vi "PH_SHS_Analysis_Statistician.PC Clear Data.vi"(0 "i ref in":refnum<vi>, 5 "error IO":errorcluster) -> (14 "i ref out":refnum<vi>, 19 "error out":errorcluster)   [LabVIEW 2014, in "PH_SHS_Analysis_Statistician.lvlib"]
uses:
  PH_SHS_Analysis_Statistician.lvlib
  PH_SHS_Analysis/PH_SHS_Analysis.Zernike Dataset.ctl
  PH_StatusHandler/PH_StatusHandler.Status.ctl
  PH_SHS_Analysis/PH_SHS_Analysis.Zernike Coefficients.ctl
  PH_Common/PH_Common.lvlib
  PH_SHS_Analysis/PH_SHS_Analysis.lvlib
  PH_StatusHandler/PH_StatusHandler.lvlib
panel:
  in  "Empty Data":T1[](array[typedef]) {"State" items=["no info", "off/false/out", "on/true/in", "Failure", "Alarm", "Status 1", "Status 2", "Status 3"]; "Zernicke Coefficients"."2nd Spherical" scale=-2.0..2.0 scale format="%.2f"; "Zernicke Coefficients"."2nd Coma y" scale=-2.0..2.0 scale format="%.2f"; "Zernicke Coefficients"."2nd Coma x" scale=-2.0..2.0 scale format="%.2f"; "Zernicke Coefficients"."2nd Astig 45°" scale=-2.0..2.0 scale format="%.2f"; "Zernicke Coefficients"."2nd Astig 0°" scale=-2.0..2.0 scale format="%.2f"; "Zernicke Coefficients"."Trefoil 30°" scale=-2.0..2.0 scale format="%.2f"; "Zernicke Coefficients"."Trefoil 0°" scale=-2.0..2.0 scale format="%.2f"; "Zernicke Coefficients"."Spherical" scale=-2.0..2.0 scale format="%.2f"; "Zernicke Coefficients"."Coma y" scale=-2.0..2.0 scale format="%.2f"; "Zernicke Coefficients"."Coma x" scale=-2.0..2.0 scale format="%.2f"; "Zernicke Coefficients"."Astig 45°" scale=-2.0..2.0 scale format="%.2f"; "Zernicke Coefficients"."Astig 0°" scale=-2.0..2.0 scale format="%.2f"; "Zernicke Coefficients"."Defocus" scale=-2.0..2.0 scale format="%.2f"; "Zernicke Coefficients"."Tilt y" scale=-2.0..2.0 scale format="%.2f"; "Zernicke Coefficients"."Tilt x" scale=-2.0..2.0 scale format="%.2f"}
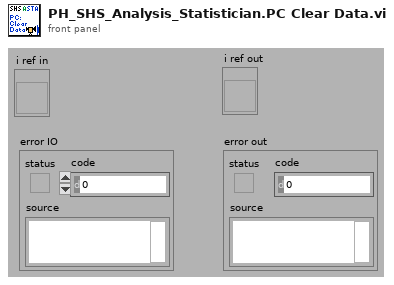
[diagram p1: front panel]
types:
  T1 = typedef "PH_SHS_Analysis.lvlib/PH_SHS_Analysis.Zernike Dataset.ctl" = cluster{"State":T2, "Time Stamp":timestamp, "PtV [lambda]":dbl, "Zernicke Coefficients":T3}
  T2 = typedef "PH_StatusHandler.lvlib/PH_StatusHandler.Status.ctl" = i16
  T3 = typedef "PH_SHS_Analysis.lvlib/PH_SHS_Analysis.Zernike Coefficients.ctl" = cluster{"Tilt x":dbl, "Tilt y":dbl, "Defocus":dbl, "Astig 0°":dbl, "Astig 45°":dbl, "Coma x":dbl, "Coma y":dbl, "Spherical":dbl, "Trefoil 0°":dbl, "Trefoil 30°":dbl, "2nd Astig 0°":dbl, "2nd Astig 45°":dbl, "2nd Coma x":dbl, "2nd Coma y":dbl, "2nd Spherical":dbl}
  T4 = typedef "PH_SHS_Analysis_Statistician.lvlib/PH_SHS_Analysis_Statistician.i attribute.ctl" = cluster{"GUI Refs ":cluster{"Status":refnum<vi>, "Result Graph":refnum<vi>, "Mean Data 1":refnum<vi>, "Std Dev Data 1":refnum<vi>, "Mean Data 2":refnum<vi>, "Std Dev Data 2":refnum<vi>, "Mean Data 3":refnum<vi>, "Std Dev Data 3":refnum<vi>, "Dummy Mean":refnum<vi>, "Dummy Std Dev":refnum<vi>, "Export Data":refnum<vi>, "Data 1":refnum<vi>, "Data 2":refnum<vi>, "Data 3":refnum<vi>, "Stat or Trend":refnum<vi>, "Delete":refnum<vi>, "Analyzer":refnum<vi>, "Current Zernike Coefficients":refnum<vi>, "PtV [Lambda]":refnum<vi>, "sample length":refnum<vi>}, "Analyzer":string, "Stat or Trend":bool, "Data 1":i16, "Data 2":i16, "Data 3":i16, "Data":T1[], "sample length":i32, "Datasets strored":i32, "Dataarray Size":i32}
  T5 = cluster{"Tilt x":dbl, "Tilt y":dbl, "Defocus":dbl, "Astig 0°":dbl, "Astig 45°":dbl, "Coma x":dbl, "Coma y":dbl, "Spherical":dbl, "Trefoil 0°":dbl, "Trefoil 30°":dbl, "2nd Astig 0°":dbl, "2nd Astig 45°":dbl, "2nd Coma x":dbl, "2nd Coma y":dbl, "2nd Spherical":dbl}
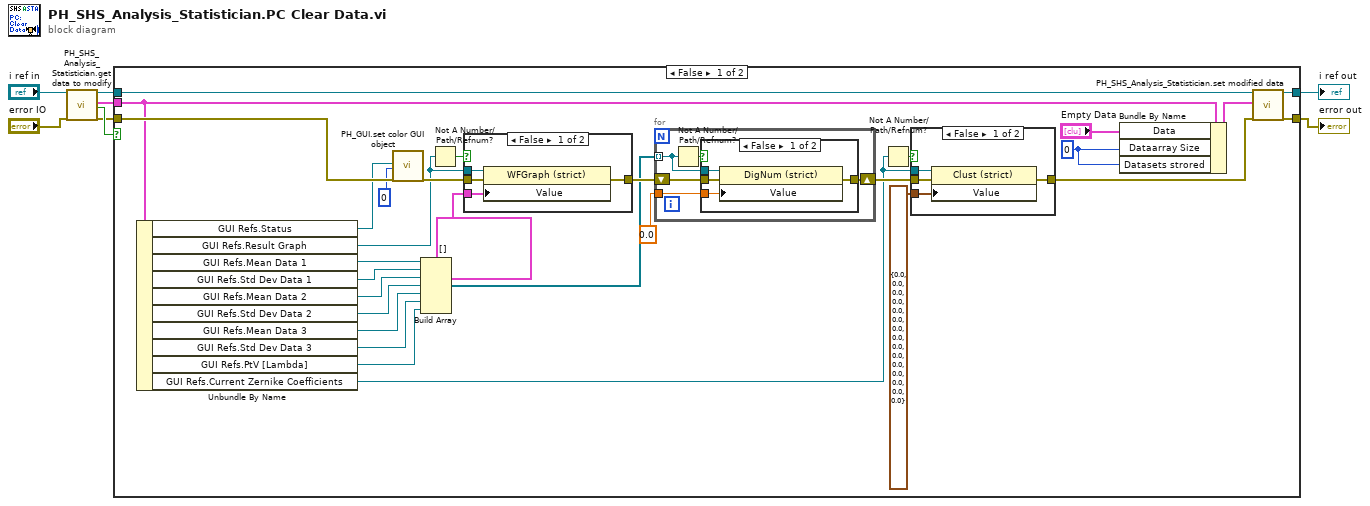
[diagram p0: block diagram]
diagram:
  n1 = call "PH_SHS_Analysis_Statistician.get data to modify.vi"("i ref in"="i ref in", "error in (no error)"="error IO") -> ("i ref out"=w5:refnum<vi>, "i attribute"=w8:T4, "timed out"=w7:bool, "error out"=w2:errorcluster)  [unwired: 14 in]
  n2 = case shown="False" w7 {
    tunnel: w2 -> [w37 w58]
    tunnel: [w36 w58] -> w3
    tunnel: w5 -> [w35 w59]
    tunnel: [w34 w59] -> w6
    tunnel: w8 -> [w31 _]
    frame False {
      w9 = 0 ("sample length")
      n3 = Unbundle By Name(w31) -> ("GUI Refs.Status"=w29:refnum<vi>, "GUI Refs.Result Graph"=w27:refnum<vi>, "GUI Refs.Mean Data 1"=w23:refnum<vi>, "GUI Refs.Std Dev Data 1"=w20:refnum<vi>, "GUI Refs.Mean Data 2"=w19:refnum<vi>, "GUI Refs.Std Dev Data 2"=w18:refnum<vi>, "GUI Refs.Mean Data 3"=w17:refnum<vi>, "GUI Refs.Std Dev Data 3"=w16:refnum<vi>, "GUI Refs.PtV [Lambda]"=w15:refnum<vi>, "GUI Refs.Current Zernike Coefficients"=w11:refnum<vi>)
      n4 = call "PH_GUI.set color GUI object.vi"("GUI object Ref"=w29, "State"=0, "error in (no error)"=w37) -> ("error out"=w30:errorcluster)  [unwired: 16 in]
      n5 = Build Array(w23, w20, w19, w18, w17, w16, w15) -> (w22:refnum<vi>[])
      n6 = Not A Number/Path/Refnum?(number/path/refnum=w27) -> (NaN/Path/Refnum?=w26:bool)
      n7 = case shown="False" w26 {
        tunnel: w30 -> [w56 w57]
        tunnel: [w55 w57] -> w24
        tunnel: w27 -> [w54 _]
        tunnel: cluster{dbl[], dbl[]}[] [] ("Value") -> [w53 _]
        frame False {
          n8 = property class="WFGraph (strict)"(reference=w54, error in=w56, "Value"=w53) -> (error out=w55:errorcluster)  [unwired: 1 out]
        }
        frame True {
        }
      }
      n9 = for {
        shift-right: [w45] -> w13
        shift-left: w24 -> [w46]
        tunnel: w22 -> [w44] mode=indexing
        tunnel: 0.0 ("Value") -> [w43]
        n10 = Not A Number/Path/Refnum?(number/path/refnum=w44) -> (NaN/Path/Refnum?=w47:bool)
        n11 = case shown="False" w47 {
          tunnel: w46 -> [w51 w52]
          tunnel: [w50 w52] -> w45
          tunnel: w44 -> [w49 _]
          tunnel: w43 -> [w48 _]
          frame False {
            n12 = property class="DigNum (strict)"(reference=w49, error in=w51, "Value"=w48) -> (error out=w50:errorcluster)  [unwired: 1 out]
          }
          frame True {
          }
        }
      }
      n13 = Not A Number/Path/Refnum?(number/path/refnum=w11) -> (NaN/Path/Refnum?=w14:bool)
      n14 = case shown="False" w14 {
        tunnel: w13 -> [w41 w42]
        tunnel: [w40 w42] -> w12
        tunnel: w11 -> [w39 _]
        tunnel: T5 {"Tilt x"=0.0, "Tilt y"=0.0, "Defocus"=0.0, "Astig 0°"=0.0, "Astig 45°"=0.0, "Coma x"=0.0, "Coma y"=0.0, "Spherical"=0.0, "Trefoil 0°"=0.0, "Trefoil 30°"=0.0, "2nd Astig 0°"=0.0, "2nd Astig 45°"=0.0, "2nd Coma x"=0.0, "2nd Coma y"=0.0, "2nd Spherical"=0.0} ("Value") -> [w38 _]
        frame False {
          n15 = property class="Clust (strict)"(reference=w39, error in=w41, "Value"=w38) -> (error out=w40:errorcluster)  [unwired: 1 out]
        }
        frame True {
        }
      }
      n16 = Bundle By Name(cluster=w31, "Data"="Empty Data", "Dataarray Size"=w9, "Datasets strored"=w9) -> (w33:T4)
      n17 = call "PH_SHS_Analysis_Statistician.set modified data.vi"("i ref in"=w35, "i attribute"=w33, "error in (no error)"=w12) -> ("i ref out"=w34:refnum<vi>, "error out"=w36:errorcluster)  [unwired: 15 in]
    }
    frame True {
    }
  }
  "i ref out" <- w6
  "error out" <- w3
